vi "showAnalysisViewer.vi"(8 "error in (no error)":errorcluster, 11 "ImageStreamViewer in":refnum<class "ImageStreamViewer.lvclass">) -> (0 "error out":errorcluster, 3 "ImageStreamViewer out":refnum<class "ImageStreamViewer.lvclass">)   [LabVIEW 2009, in "Views.lvlib" / "Camera.lvlib" / "ImageStreamViewer.lvclass"]
uses:
  ImageStreamViewer.lvclass
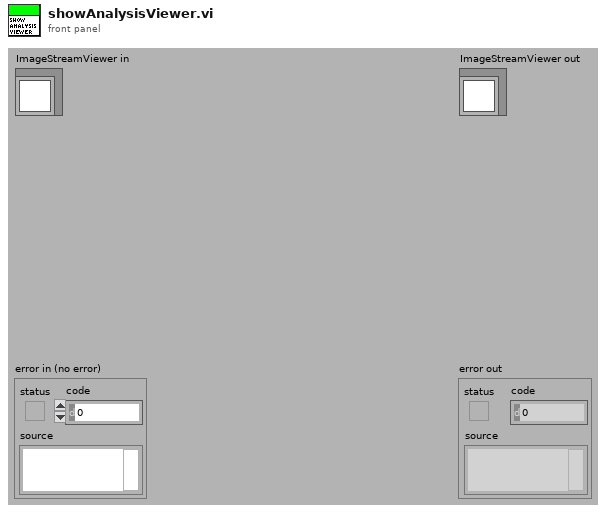
[diagram p1: front panel]
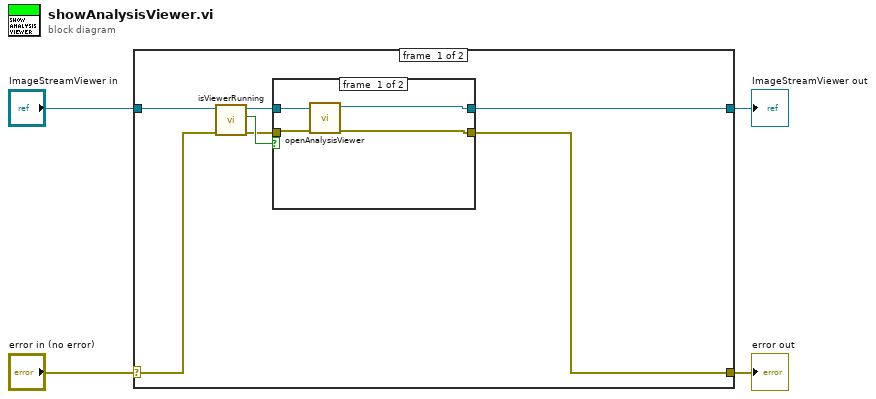
[diagram p0: block diagram]
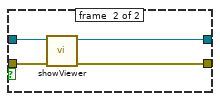
[diagram p2: hidden frame]
diagram:
  n1 = case shown="No Error" "error in (no error)" {
    selector: "error in (no error)" -> [w10 w21]
    tunnel: [w5 w21] -> w3
    tunnel: [w6 w20] -> w1
    tunnel: "ImageStreamViewer in" -> [w11 w20]
    frame #0 {
      n2 = call "isViewerRunning.vi"("error in (no error)"=w10, "ImageStreamViewer in"=w11) -> ("error out"=w8:errorcluster, "running?"=w9:bool, "ImageStreamViewer out"=w7:refnum<class "ImageStreamViewer.lvclass">)  [unwired: 7 in]
      n3 = case shown="False" w9 {
        tunnel: w8 -> [w14 w18]
        tunnel: w7 -> [w15 w19]
        tunnel: [w13 w17] -> w6
        tunnel: [w12 w16] -> w5
        frame #0 {
          n4 = call "openAnalysisViewer.vi"("error in (no error)"=w14, "ImageStreamViewer in"=w15) -> ("error out"=w12:errorcluster, "ImageStreamViewer out"=w13:refnum<class "ImageStreamViewer.lvclass">)  [unwired: 8 in]
        }
        frame #1 {
          n5 = call "showViewer.vi"("error in (no error)"=w18, "ImageStreamViewer in"=w19) -> ("error out"=w16:errorcluster, "ImageStreamViewer out"=w17:refnum<class "ImageStreamViewer.lvclass">)  [unwired: 8 in]
        }
      }
    }
    frame #1 {
    }
  }
  "error out" <- w3
  "ImageStreamViewer out" <- w1
